vi "Roll state (SubVI).vi"(9 "# each state":i32[](array[numeric])=[100, 60, 2], 11 "Unrolled state":i32) -> (3 "State array":i32[](array[numeric]))   [LabVIEW 2013]
doc: "Unrolls an N-dimension array to a 1D array so that it can be processed by the Q-learning algorithm.\n\nE.g. A 3 x 5 array is unrolled to a 15 x 1 array."
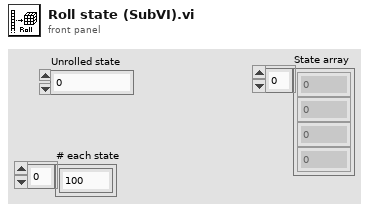
[diagram p1: front panel]
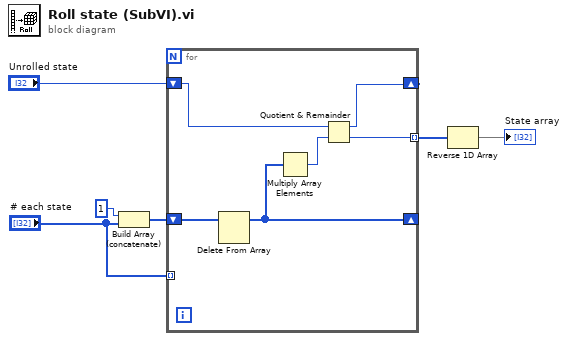
[diagram p0: block diagram]
diagram:
  n1 = Build Array (concatenate)(1, "# each state") -> (w5:i32[])
  n2 = for {
    shift-right: [w10] -> _
    shift-left: w5 -> [w12]
    tunnel: [w9] -> w3 mode=indexing
    tunnel: "# each state" -> [_] mode=indexing
    shift-right: [w8] -> _
    shift-left: "Unrolled state" -> [w7]
    n3 = Delete From Array(array=w12) -> (array with subset deleted=w10:i32[])  [unwired: 2 in, 1 out]
    n4 = Multiply Array Elements(1:w10) -> (0:w11:i32)
    n5 = Quotient & Remainder(x=w7, y=w11) -> (x-y*floor(x/y)=w8:i32, floor(x/y)=w9:i32)
  }
  n6 = Reverse 1D Array(array=w3) -> (reversed array=→"State array":i32[])
